vi "Points Difference.vi"(1 "Nb de points (boucle consommatrice)":i32, 2 "Refnum de la commande Points manqués":refnum<vi>, 3 "Nb de points (boucle productrice)":i32) -> (0 "Points manqués":i32)   [LabVIEW 2009]
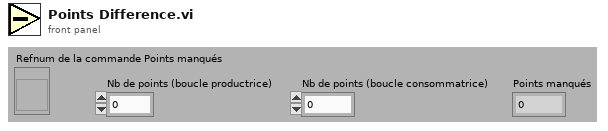
[diagram p1: front panel]
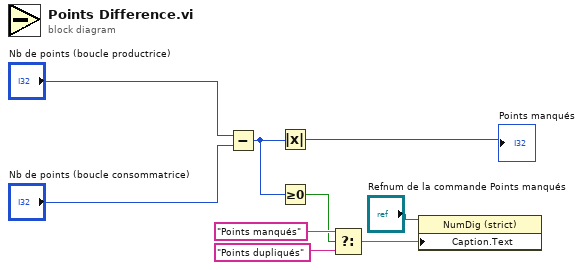
[diagram p0: block diagram]
diagram:
  n1 = Subtract(x="Nb de points (boucle productrice)", y="Nb de points (boucle consommatrice)") -> (x-y=w8:i32)
  n2 = Absolute Value(x=w8) -> (abs(x)=→"Points manqués":i32)
  n3 = Greater Or Equal To 0?(x=w8) -> (x >= 0?=w4:bool)
  n4 = Select(t="Points manqués", s=w4, f="Points dupliqués") -> (s? t:f=w7:string)
  n5 = property on="Property Node" class="NumDig (strict)"(reference="Refnum de la commande Points manqués", "Caption.Text"=w7) -> ()  [unwired: 1 in, 2 out]
